vi "数据处理直接插入整合 (子VI).vi"   [LabVIEW 2016, in "数据传输系统.lvlib"]
types:
  T1 = cluster{"PH":string[][], "CODCr":string[][], "氨氮":string[][], "CODMn":string[][], "总氮":string[][], "总磷":string[][], "电导率":string[][], "水温":string[][], "DO":string[][], "浊度":string[][], "叶绿素":string[][], "藻密度":string[][], "铜":string[][], "盐度":string[][], "水位":string[][], "流速":string[][], "瞬时流量":string[][], "累积流量":string[][], "亚硝酸盐":string[][], "硫化物":string[][], "ORP":string[][], "铅":string[][], "镉":string[][], "锌":string[][], "镍":string[][], "锰":string[][], "汞":string[][], "气温":string[][], "气压":string[][], "风速":string[][], "风向":string[][]}
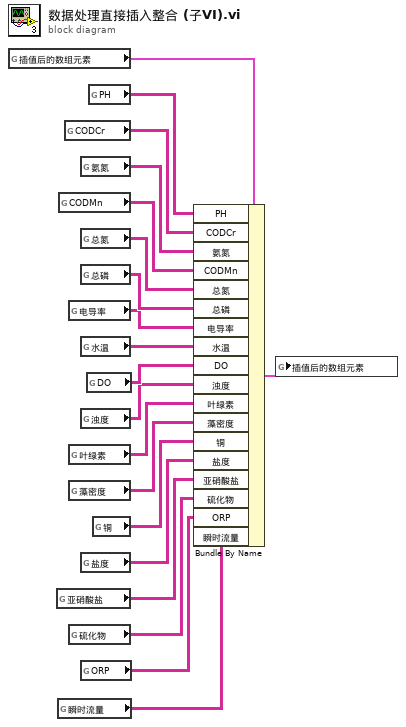
[diagram p0: block diagram]
diagram:
  n1 = global read "插值后的新数组.vi" "插值后的数组元素"() -> (w6:T1)
  n2 = global read "全局 所有参数.vi" "亚硝酸盐"() -> (w3:string[][])
  n3 = global read "全局 所有参数.vi" "瞬时流量"() -> (w1:string[][])
  n4 = global read "全局 所有参数.vi" "CODMn"() -> (w17:string[][])
  n5 = global read "全局 所有参数.vi" "CODCr"() -> (w19:string[][])
  n6 = global read "全局 所有参数.vi" "电导率"() -> (w14:string[][])
  n7 = global read "全局 所有参数.vi" "叶绿素"() -> (w10:string[][])
  n8 = global read "全局 所有参数.vi" "藻密度"() -> (w9:string[][])
  n9 = global read "全局 所有参数.vi" "硫化物"() -> (w4:string[][])
  n10 = global read "全局 所有参数.vi" "氨氮"() -> (w18:string[][])
  n11 = global read "全局 所有参数.vi" "总氮"() -> (w16:string[][])
  n12 = global read "全局 所有参数.vi" "总磷"() -> (w15:string[][])
  n13 = global read "全局 所有参数.vi" "水温"() -> (w13:string[][])
  n14 = global read "全局 所有参数.vi" "浊度"() -> (w11:string[][])
  n15 = global read "全局 所有参数.vi" "盐度"() -> (w7:string[][])
  n16 = global read "全局 所有参数.vi" "ORP"() -> (w5:string[][])
  n17 = global read "全局 所有参数.vi" "DO"() -> (w12:string[][])
  n18 = global read "全局 所有参数.vi" "PH"() -> (w20:string[][])
  n19 = global read "全局 所有参数.vi" "铜"() -> (w8:string[][])
  n20 = Bundle By Name(cluster=w6, "PH"=w20, "CODCr"=w19, "氨氮"=w18, "CODMn"=w17, "总氮"=w16, "总磷"=w15, "电导率"=w14, "水温"=w13, "DO"=w12, "浊度"=w11, "叶绿素"=w10, "藻密度"=w9, "铜"=w8, "盐度"=w7, "亚硝酸盐"=w3, "硫化物"=w4, "ORP"=w5, "瞬时流量"=w1) -> (w2:T1)
  n21 = global write "插值后的新数组.vi" "插值后的数组元素"(w2) -> ()
